vi "convert-dev-to-json.vi"(8 "添加空调":bool, 11 "dev-cmd-list":T1(array[cluster])) -> (0 "LV Text":string, 3 "<JSON>":string caption="<JSON>Object")   [LabVIEW 2019]
uses:
  e439d0ca-603d-4de6-9a28-db9d424adf78.vi
  29729271-875d-4357-8c55-ac745915a45a.vi
  <vilib>/JDP Science/JSONtext/support/Format JSON Object.vi
  <vilib>/JDP Science/JSONtext/Variant to JSON Text.vi
  <vilib>/JDP Science/JSONtext/Get all Object Items.vi
  <vilib>/JDP Science/JSONtext/Set Multiple Object Items.vi
  <vilib>/JDP Science/JSONtext/JSONtext.lvlib
  <vilib>/addons/Tools/Unicode/UTF8 Tools.lvlib
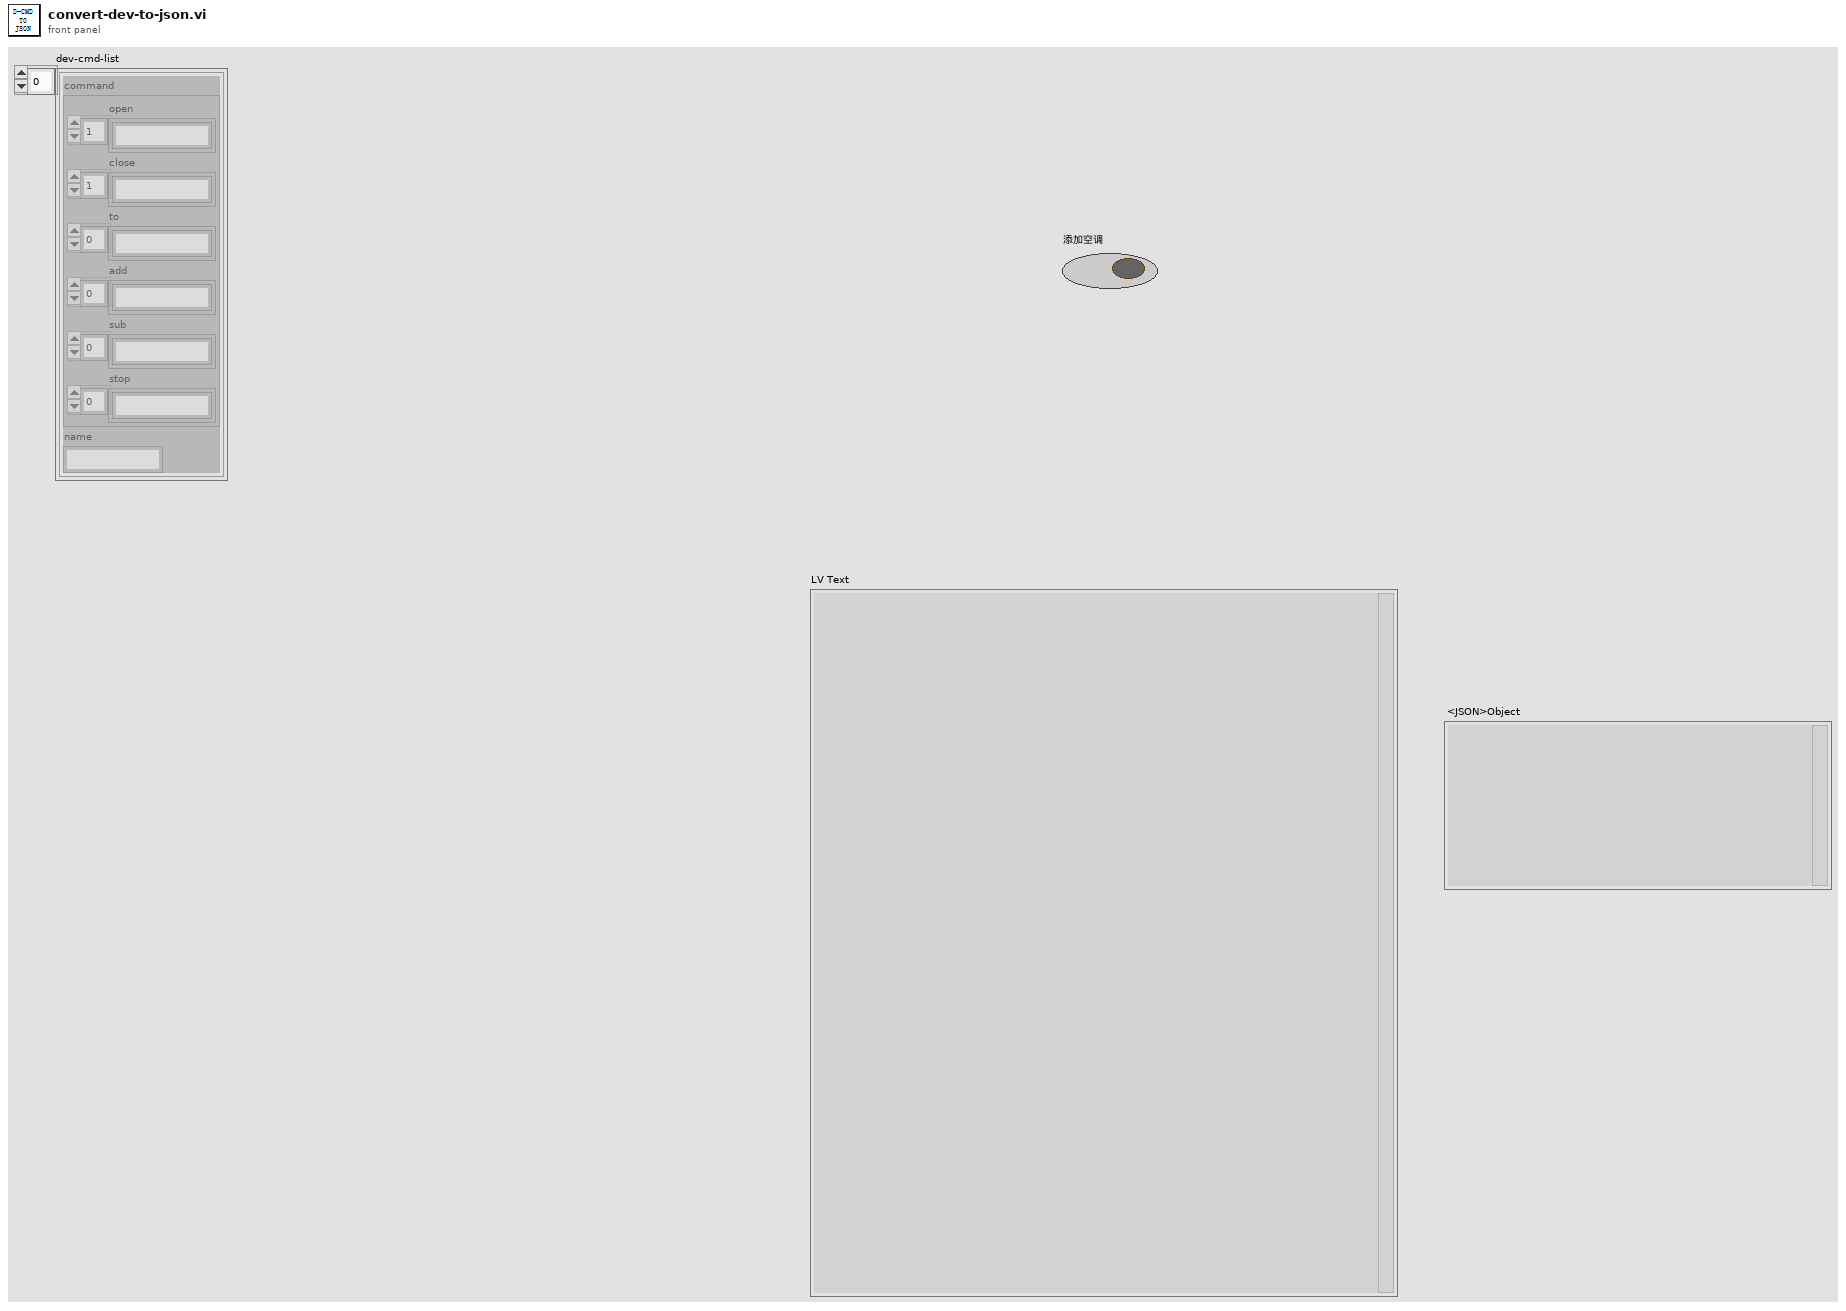
[diagram p1: front panel]
types:
  T1 = cluster{"command":cluster{"open":string[], "close":string[], "to":string[], "add":string[], "sub":string[], "stop":string[]}, "name":string}[]
  T2 = cluster{"open":string[], "close":string[], "to":string[], "add":string[], "sub":string[], "stop":string[]}
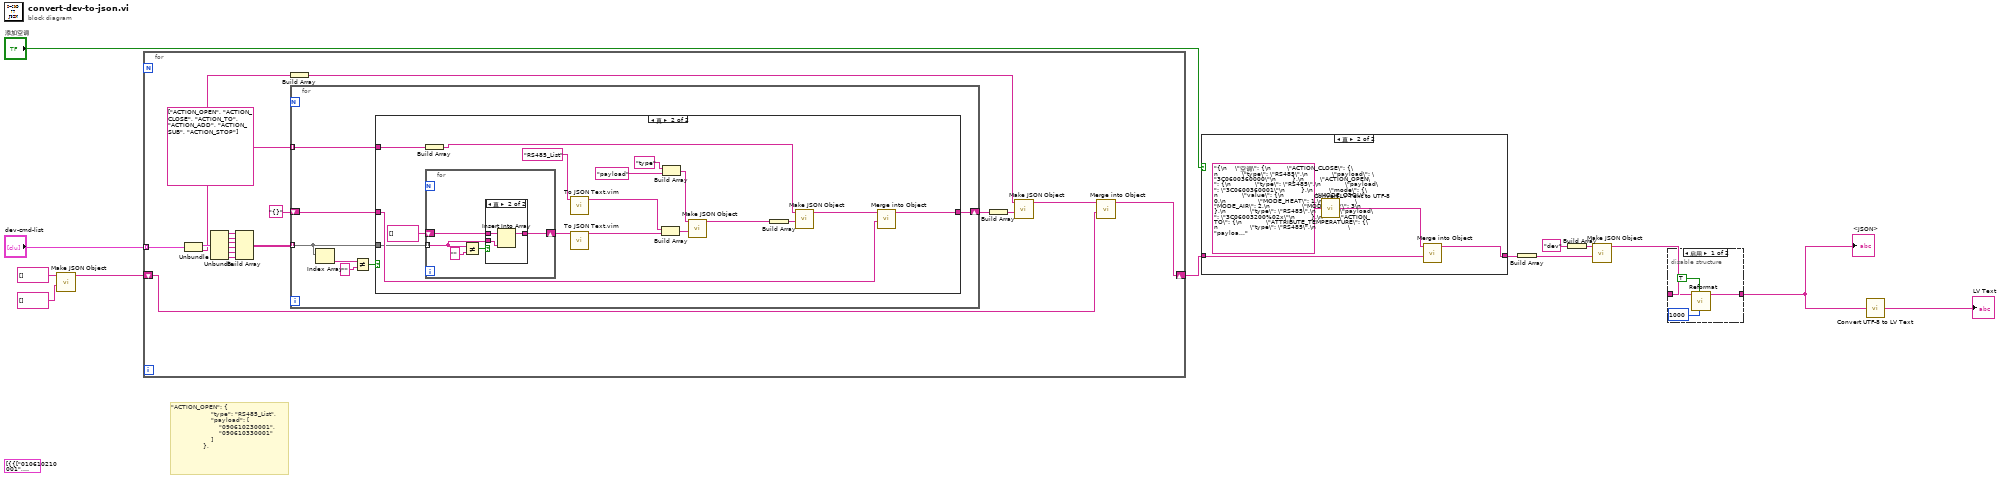
[diagram p0: block diagram]
diagram:
  (unwired) T1 [{"command"={"open"=["010610210001", "010610310001"], "close"=["010610210000", "010610310000"], "to"=[], "add"=[], "sub"=[], "stop"=[]}, "name"="水电费"}, {"command"={"open"=["010610210001", "010610310001"], "close"=["010610210000", "010610310000"], "to"=[], "add"=[], "sub"=[], "stop"=[]}, "name"="温柔"}, {"command"={"open"=["010610210001", "010610310001"], "close"=["010610210000", "010610310000"], "to"=[], "add"=[], "sub"=[], "stop"=[]}, "name"="许"}] ("dev-cmd-list")
  # "\"ACTION_OPEN\": {\n                    \"type\": \"RS485_List\",\n                    \"payload\": [\n                        \"090610230001\",\n                        \"090610330001\"\n                    ]\n                },"
  n1 = call <vilib>:"Make JSON Object.vi"("JSON Items"=string[] [], "Item Names"=string[] []) -> ("<JSON>"=w10:string)  [unwired: 8 in, 1 out]
  n2 = for {
    tunnel: "dev-cmd-list" -> [w31] mode=indexing
    shift-right: [w15] -> w4
    shift-left: w10 -> [w14]
    n3 = Unbundle(w31) -> ("command"=w30:T2, "name"=w20:string)
    n4 = Unbundle(w30) -> ("open"=w28:string[], "close"=w27:string[], "to"=w26:string[], "add"=w25:string[], "sub"=w24:string[], "stop"=w23:string[])
    n5 = Build Array(w28, w27, w26, w25, w24, w23) -> (w22:string[][])
    n6 = Build Array(w20) -> (w19:string[])
    n7 = for {
      tunnel: string[] ["ACTION_OPEN", "ACTION_CLOSE", "ACTION_TO", "ACTION_ADD", "ACTION_SUB", "ACTION_STOP"] ("open") -> [w38] mode=indexing
      tunnel: w22 -> [w35] mode=indexing
      shift-right: [w36] -> w18
      shift-left: "{}" ("<JSON>") -> [w37]
      n8 = Index Array(array=w35) -> (element=w34:string)  [unwired: 1 in]
      n9 = Not Equal?(x=w34, y="") -> (x != y?=w32:bool)
      n10 = case shown="真" w32 {
        tunnel: w38 -> [_ w50]
        tunnel: w37 -> [w39 w45]
        tunnel: [w39 w44] -> w36
        tunnel: w35 -> [_ w43]
        frame False {
        }
        frame True {
          n11 = Build Array(w50) -> (w47:string[])
          n12 = for {
            tunnel: w43 -> [w59] mode=indexing
            shift-right: [w57] -> w41
            shift-left: string[] [] -> [w58]
            n13 = Not Equal?(x=w59, y="") -> (x != y?=w60:bool)
            n14 = case shown="真" w60 {
              tunnel: w59 -> [_ w64]
              tunnel: w58 -> [w62 w65]
              tunnel: [w62 w63] -> w57
              frame False {
              }
              frame True {
                n15 = Insert Into Array(array=w65, new element=w64) -> (w63:string[])  [unwired: 1 in]
              }
            }
          }
          n16 = call "To JSON Text.vim"("Anything"="RS485_List") -> ("<JSON>"=w55:string)  [unwired: 9 in, 1 out]
          n17 = call "To JSON Text.vim"("Anything"=w41) -> ("<JSON>"=w40:string)  [unwired: 9 in, 1 out]
          n18 = Build Array(w55, w40) -> (w56:string[])
          n19 = Build Array("type", "payload") -> (w54:string[])
          n20 = call <vilib>:"Make JSON Object.vi"("JSON Items"=w56, "Item Names"=w54) -> ("<JSON>"=w49:string)  [unwired: 8 in, 1 out]
          n21 = Build Array(w49) -> (w48:string[])
          n22 = call <vilib>:"Make JSON Object.vi"("JSON Items"=w48, "Item Names"=w47) -> ("<JSON>"=w46:string)  [unwired: 8 in, 1 out]
          n23 = call <vilib>:"Merge into Object.vi"("JSON Object to Merge"=w45, "JSON"=w46) -> ("<JSON>"=w44:string)  [unwired: 7 in, 1 out]
        }
      }
    }
    n24 = Build Array(w18) -> (w17:string[])
    n25 = call <vilib>:"Make JSON Object.vi"("JSON Items"=w17, "Item Names"=w19) -> ("<JSON>"=w16:string)  [unwired: 8 in, 1 out]
    n26 = call <vilib>:"Merge into Object.vi"("JSON Object to Merge"=w14, "JSON"=w16) -> ("<JSON>"=w15:string)  [unwired: 7 in, 1 out]
  }
  n27 = case shown="真" "添加空调" {
    tunnel: w4 -> [w66 w70]
    tunnel: [w66 w67] -> w2
    frame False {
    }
    frame True {
      n28 = call <vilib>:"Convert LV Text to UTF-8.vi"("LV Text"="{\n    \"空调\": {\n        \"ACTION_CLOSE\": {\n            \"type\": \"RS485\",\n            \"payload\": \"3C0600360000\"\n        },\n        \"ACTION_OPEN\": {\n            \"type\": \"RS485\",\n            \"payload\": \"3C0600360001\"\n        },\n        \"mode\": {\n            \"value\": {\n                \"MODE_COOL\": 0,\n                \"MODE_HEAT\": 1,\n                \"MODE_AIR\": 2,\n                \"MODE_DRY\": 3\n            },\n            \"type\": \"RS485\",\n            \"payload\": \"3C06003200%02x\"\n        },\n        \"ACTION_TO\": {\n            \"ATTRIBUTE_TEMPERATURE\": {\n                \"type\": \"RS485\",\n                \"payload\": \"3C06003500%02x\"\n            },\n            \"ATTRIBUTE_WIND_SPEED\": {\n                \"value\": {\n                    \"VALUE_LOW\": 1,\n                    \"VALUE_MIDDLE\": 2,\n                    \"VALUE_HIGH\": 3,\n                    \"VALUE_AUTO\": 4\n                },\n                \"type\": \"RS485\",\n                \"payload\": \"3C06003300%02x\"\n            }\n        },\n        \"ACTION_ADD\": {\n            \"ATTRIBUTE_TEMPERATURE\": {\n                \"type\": \"RS485\",\n                \"payload\": \"addd12445a\"\n            }\n        },\n        \"ACTION_REDUCE\": {\n            \"ATTRIBUTE_TEMPERATURE\": {\n                \"type\": \"RS485\",\n                \"payload\": \"ddd5644e21\"\n            }\n        }\n    }\n}") -> ("UTF-8 Text"=w68:string)  [unwired: 13 in, 1 out]
      n29 = call <vilib>:"Merge into Object.vi"("JSON Object to Merge"=w70, "JSON"=w68) -> ("<JSON>"=w67:string)  [unwired: 7 in, 1 out]
    }
  }
  n30 = Build Array(w2) -> (w8:string[])
  n31 = Build Array("dev") -> (w7:string[])
  n32 = call <vilib>:"Make JSON Object.vi"("JSON Items"=w8, "Item Names"=w7) -> ("<JSON>"=w5:string)  [unwired: 8 in, 1 out]
  n33 = disable-structure shown="启用" {
    disable-tunnel: w5 -> [w74 w75]
    disable-tunnel: [w73 w75] -> w1
    frame Enabled {
      n34 = call <vilib>:"Reformat.vi"("Pretty Print Levels"=1000, "Alphabetically Sort Objects"=TRUE, "JSON"=w74) -> ("<JSON>First JSON Value\n\n<JSON>"=w73:string)  [unwired: 5 in, 3 out]
    }
    frame Disabled {
    }
  }
  "<JSON>" <- w1
  n35 = call <vilib>:"Convert UTF-8 to LV Text.vi"("UTF-8 Text"=w1) -> ("LV Text"=→"LV Text":string)  [unwired: 13 in, 1 out]
